vi "SerialReadWrite.vi"() -> ()   [LabVIEW 2020]
uses:
  <vilib>/Instr/_visa.llb/VISA Configure Serial Port (Instr).vi
panel:
  in  "Start":bool
  in  "stop":bool
  out "?":bool
  out "?":bool
  out "?":bool
  out "?":bool
  out "?":bool
  out "?":bool
  in  "Color":string(combo)
  in  "LED No":string(combo)
  out "Read Data":string
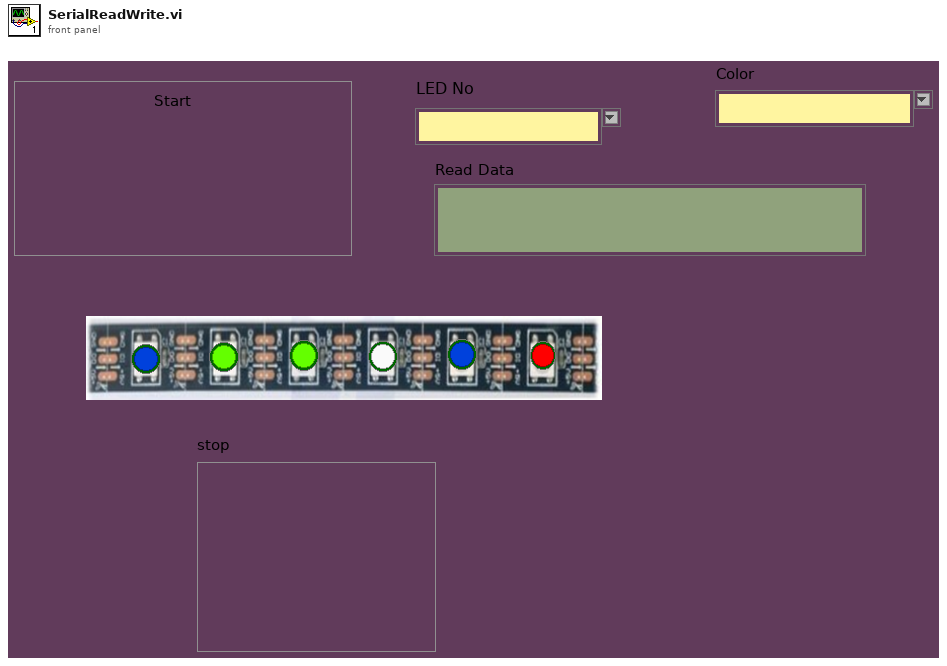
[diagram p1: front panel]
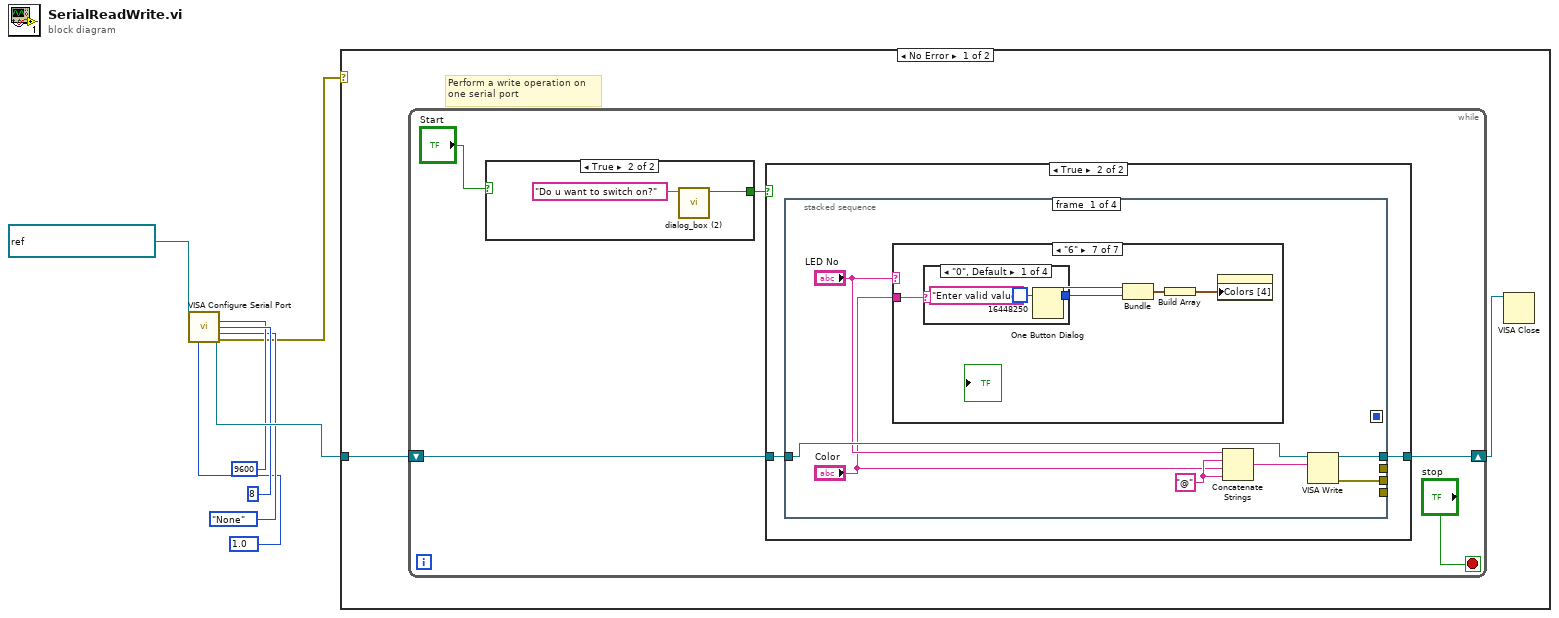
[diagram p0: block diagram]
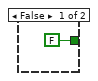
[diagram p2: hidden frame]
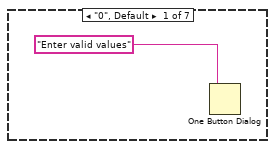
[diagram p4: hidden frame]
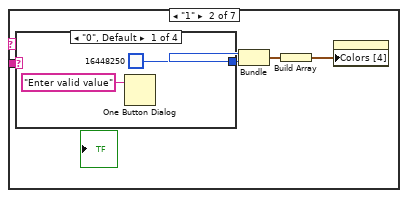
[diagram p5: hidden frame]
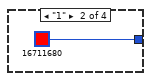
[diagram p6: hidden frame]
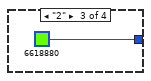
[diagram p7: hidden frame]
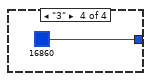
[diagram p8: hidden frame]
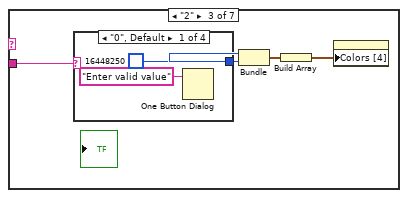
[diagram p9: hidden frame]
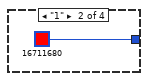
[diagram p10: hidden frame]
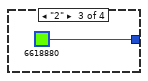
[diagram p11: hidden frame]
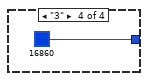
[diagram p12: hidden frame]
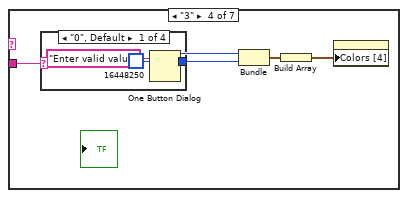
[diagram p13: hidden frame]
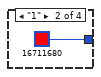
[diagram p14: hidden frame]
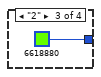
[diagram p15: hidden frame]
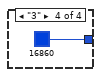
[diagram p16: hidden frame]
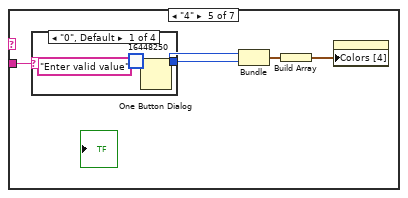
[diagram p17: hidden frame]
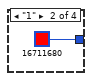
[diagram p18: hidden frame]
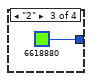
[diagram p19: hidden frame]
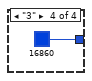
[diagram p20: hidden frame]
diagram:
  w2 = u16 10 items=["1.0"=10, "1.5"=15, "2.0"=20] ("stop bits (10: 1 bit)")
  n1 = call-poly "VISA Configure Serial Port"("VISA resource name"=refnum<visa-resource-name> "COM3", "baud rate (9600)"=u32 9600, "data bits (8)"=u16 8, "parity (0:none)"=enum16{"None", "Odd", "Even", "Mark", "Space"}."None", "stop bits (10: 1 bit)"=w2) -> ("VISA resource name out"=w7:refnum<visa-resource-name>, "error out"=w1:errorcluster)  [unwired: 4 in, 5 out]
  n2 = case shown="No Error" w1 {
    tunnel: w7 -> [w9 _]
    frame No Error {
      # "Perform a write operation on one serial port"
      n3 = while {
        shift-right: [w13] -> w8
        shift-left: w9 -> [w14]
        stop <- "stop" stop-if-true
        n4 = case shown="True" "Start" {
          tunnel: [FALSE w17] -> w12
          frame False {
          }
          frame True {
            n5 = call "dialog_box (2).vi"("INPUT"="Do u want to switch on?") -> ("Boolean"=w17:bool)  [unwired: 9 in]
          }
        }
        n6 = case shown="True" w12 {
          tunnel: w14 -> [w18 w20]
          tunnel: [w18 w19] -> w13
          frame False {
          }
          frame True {
            n7 = stacked-sequence {
              seq-local: [_ _ w85 _] -> [_ _ _ w89]
              tunnel: w20 -> [w27 _ w86 w90]
              tunnel: [w26 _ _ _] -> w19
              tunnel: [w25 _ _ _] -> _
              tunnel: [_ _ _ w88] -> _
              tunnel: [_ _ w84 _] -> _
              frame #0 {
                w23 = "@" ("string")
                n8 = case shown="\"6\"" "LED No" {
                  tunnel: "Color" -> [_ w29 w38 w47 w56 w65 w74]
                  frame "0", Default {
                    n9 = One Button Dialog(message="Enter valid values") -> ()  [unwired: 1 in, 1 out]
                  }
                  frame "1" {
                    n10 = case shown="\"0\", Default" w29 {
                      tunnel: [u32 16448250 u32 16711680 u32 6618880 u32 16860] -> w32
                      frame "0", Default {
                        n11 = One Button Dialog(message="Enter valid value") -> ()  [unwired: 1 in, 1 out]
                      }
                      frame "1" {
                      }
                      frame "2" {
                      }
                      frame "3" {
                      }
                    }
                    n12 = Bundle(w32, w32) -> (w31:cluster{u32, u32})  [unwired: 1 in]
                    n13 = Build Array(w31) -> (w30:cluster{u32, u32}[])
                    n14 = property class="Bool (strict)"("Colors [4]"=w30) -> ()  [unwired: 2 in, 2 out]
                  }
                  frame "2" {
                    n15 = case shown="\"0\", Default" w38 {
                      tunnel: [u32 16448250 u32 16711680 u32 6618880 u32 16860] -> w39
                      frame "0", Default {
                        n16 = One Button Dialog(message="Enter valid value") -> ()  [unwired: 1 in, 1 out]
                      }
                      frame "1" {
                      }
                      frame "2" {
                      }
                      frame "3" {
                      }
                    }
                    n17 = Bundle(w39, w39) -> (w40:cluster{u32, u32})  [unwired: 1 in]
                    n18 = Build Array(w40) -> (w41:cluster{u32, u32}[])
                    n19 = property class="Bool (strict)"("Colors [4]"=w41) -> ()  [unwired: 2 in, 2 out]
                  }
                  frame "3" {
                    n20 = case shown="\"0\", Default" w47 {
                      tunnel: [u32 16448250 u32 16711680 u32 6618880 u32 16860] -> w50
                      frame "0", Default {
                        n21 = One Button Dialog(message="Enter valid value") -> ()  [unwired: 1 in, 1 out]
                      }
                      frame "1" {
                      }
                      frame "2" {
                      }
                      frame "3" {
                      }
                    }
                    n22 = Bundle(w50, w50) -> (w49:cluster{u32, u32})  [unwired: 1 in]
                    n23 = Build Array(w49) -> (w48:cluster{u32, u32}[])
                    n24 = property class="Bool (strict)"("Colors [4]"=w48) -> ()  [unwired: 2 in, 2 out]
                  }
                  frame "4" {
                    n25 = case shown="\"0\", Default" w56 {
                      tunnel: [u32 16448250 u32 16711680 u32 6618880 u32 16860] -> w59
                      frame "0", Default {
                        n26 = One Button Dialog(message="Enter valid value") -> ()  [unwired: 1 in, 1 out]
                      }
                      frame "1" {
                      }
                      frame "2" {
                      }
                      frame "3" {
                      }
                    }
                    n27 = Bundle(w59, w59) -> (w58:cluster{u32, u32})  [unwired: 1 in]
                    n28 = Build Array(w58) -> (w57:cluster{u32, u32}[])
                    n29 = property class="Bool (strict)"("Colors [4]"=w57) -> ()  [unwired: 2 in, 2 out]
                  }
                  frame "5" {
                    n30 = case shown="\"0\", Default" w65 {
                      tunnel: [u32 16448250 u32 16711680 u32 6618880 u32 16860] -> w66
                      frame "0", Default {
                        n31 = One Button Dialog(message="Enter valid value") -> ()  [unwired: 1 in, 1 out]
                      }
                      frame "1" {
                      }
                      frame "2" {
                      }
                      frame "3" {
                      }
                    }
                    n32 = Bundle(w66, w66) -> (w67:cluster{u32, u32})  [unwired: 1 in]
                    n33 = Build Array(w67) -> (w68:cluster{u32, u32}[])
                    n34 = property class="Bool (strict)"("Colors [4]"=w68) -> ()  [unwired: 2 in, 2 out]
                  }
                  frame "6" {
                    n35 = case shown="\"0\", Default" w74 {
                      tunnel: [u32 16448250 u32 16711680 u32 6618880 u32 16860] -> w75
                      frame "0", Default {
                        n36 = One Button Dialog(message="Enter valid value") -> ()  [unwired: 1 in, 1 out]
                      }
                      frame "1" {
                      }
                      frame "2" {
                      }
                      frame "3" {
                      }
                    }
                    n37 = Bundle(w75, w75) -> (w76:cluster{u32, u32})  [unwired: 1 in]
                    n38 = Build Array(w76) -> (w77:cluster{u32, u32}[])
                    n39 = property class="Bool (strict)"("Colors [4]"=w77) -> ()  [unwired: 2 in, 2 out]
                  }
                }
                n40 = Concatenate Strings("LED No", w23, "Color", w23) -> (w24:string)
                n41 = VISA Write(VISA resource name=w27, write buffer=w24) -> (VISA resource name out=w26:refnum<visa-resource-name>, error out=w25:errorcluster)  [unwired: 1 in, 1 out]
              }
              frame #1 {
                n42 = Wait (ms)(milliseconds to wait=u32 100 ("millisecond timer value")) -> ()  [unwired: 1 out]
              }
              frame #2 {
                n43 = property class="Instr"(reference=w86) -> (error out=w84:errorcluster, "Bytes at Port"=w85:u32)  [unwired: 1 in, 1 out]
              }
              frame #3 {
                n44 = VISA Read(VISA resource name=w90, byte count=w89) -> (read buffer=→"Read Data":string, error out=w88:errorcluster)  [unwired: 1 in, 2 out]
              }
            }
          }
        }
      }
      n45 = VISA Close(VISA resource name=w8) -> ()  [unwired: 1 in, 1 out]
    }
    frame Error {
      n46 = One Button Dialog(message="Check COM") -> ()  [unwired: 1 in, 1 out]
    }
  }
